vi "Configure Inputs.vi"(0 "VISA resource name":refnum<visa-resource-name>, 1 "Coupling (0: cplAC)":i32(ring) items=["cplAC", "cplDC"], 2 "Auto Range Input (T: Enable)":bool=TRUE, 3 "Enable Termination (T: Enable)":bool=TRUE, 5 "Domain (0: idAnalog)":i32(ring) items=["idAnalog", "idDigital", "idGenMon"], 7 "Channels (1)":i32=1, 9 "Connector Type (0: cXLR)":i32(ring) items=["cXLR", "cBNC", "cOptical"], 11 "error in (no error)":errorcluster, 12 "Analog Bandwidth (0: bw200kHz)":i32(ring) items=["bw200kHz", "bw50kHz", "bw25kHz"], 13 "Enable Digital Dual Connector (T: Enable)":bool=TRUE) -> (4 "VISA resource name out":refnum<visa-resource-name>, 15 "error out":errorcluster)   [LabVIEW 2014, in "Stanford Research SR1.lvlib"]
doc: "Configures the attributes for the Quick Measurement Inputs."
uses:
  Stanford Research SR1.lvlib
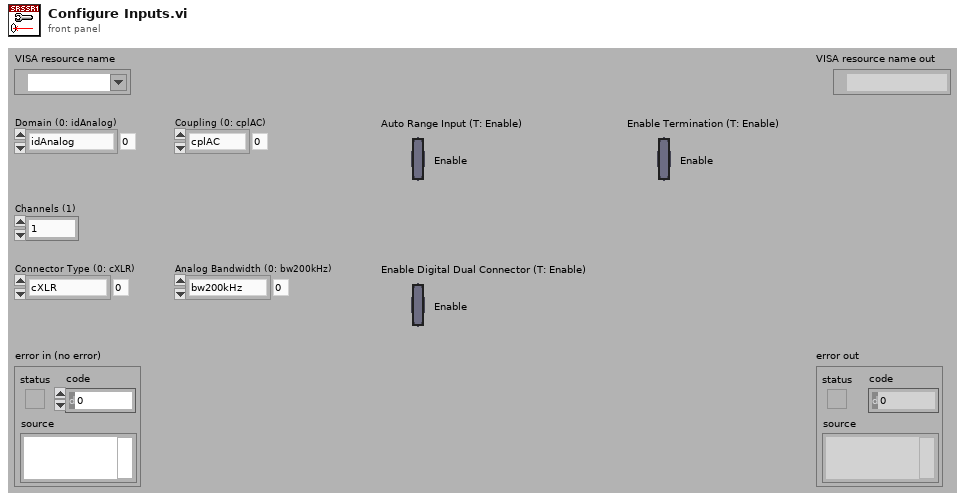
[diagram p1: front panel]
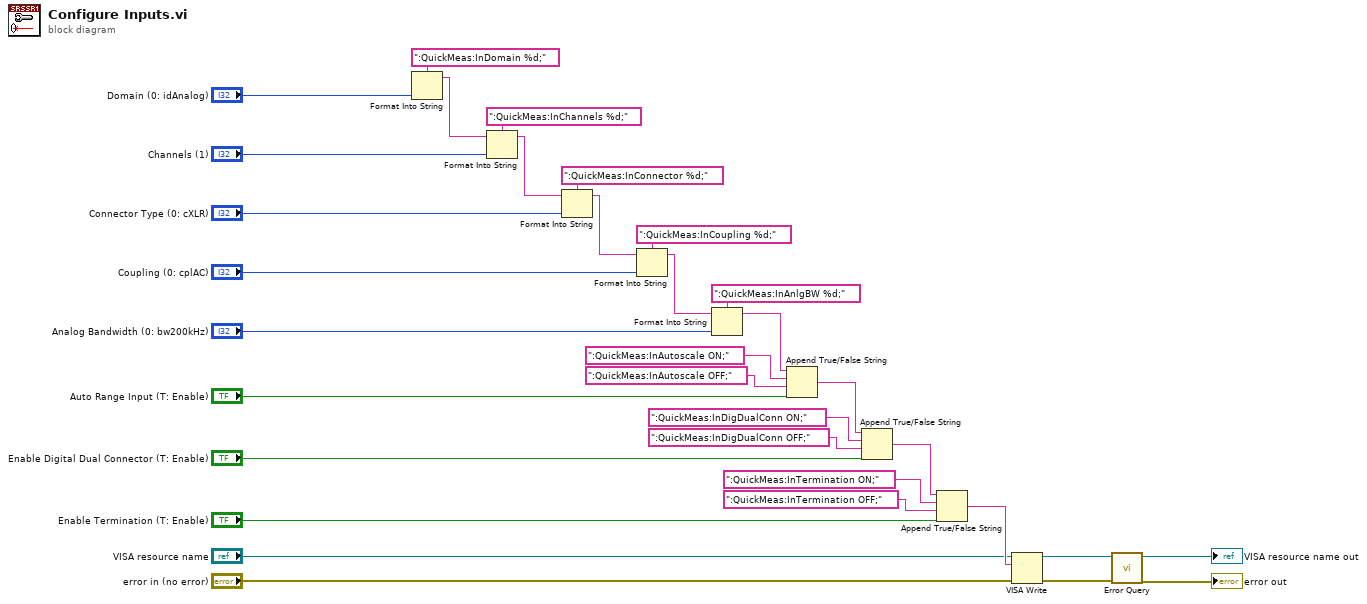
[diagram p0: block diagram]
diagram:
  n1 = Format Into String(format string=":QuickMeas:InDomain %d;", "Domain (0: idAnalog)") -> (resulting string=w31:string)  [unwired: 2 in, 1 out]
  n2 = Format Into String(format string=":QuickMeas:InChannels %d;", initial string=w31, "Channels (1)") -> (resulting string=w28:string)  [unwired: 1 in, 1 out]
  n3 = Format Into String(format string=":QuickMeas:InConnector %d;", initial string=w28, "Connector Type (0: cXLR)") -> (resulting string=w25:string)  [unwired: 1 in, 1 out]
  n4 = Format Into String(format string=":QuickMeas:InCoupling %d;", initial string=w25, "Coupling (0: cplAC)") -> (resulting string=w22:string)  [unwired: 1 in, 1 out]
  n5 = Format Into String(format string=":QuickMeas:InAnlgBW %d;", initial string=w22, "Analog Bandwidth (0: bw200kHz)") -> (resulting string=w19:string)  [unwired: 1 in, 1 out]
  n6 = Append True/False String(1:"Auto Range Input (T: Enable)", 2:":QuickMeas:InAutoscale OFF;", 3:":QuickMeas:InAutoscale ON;", 4:w19) -> (0:w15:string)
  n7 = Append True/False String(1:"Enable Digital Dual Connector (T: Enable)", 2:":QuickMeas:InDigDualConn OFF;", 3:":QuickMeas:InDigDualConn ON;", 4:w15) -> (0:w11:string)
  n8 = Append True/False String(1:"Enable Termination (T: Enable)", 2:":QuickMeas:InTermination OFF;", 3:":QuickMeas:InTermination ON;", 4:w11) -> (0:w7:string)
  n9 = VISA Write(VISA resource name="VISA resource name", write buffer=w7, error in (no error)="error in (no error)") -> (VISA resource name out=w4:refnum<visa-resource-name>, error out=w3:errorcluster)  [unwired: 1 out]
  n10 = call "Error Query.vi"("error in (no error)"=w3, "VISA resource name"=w4) -> ("error out"=→"error out":errorcluster, "VISA resource name out"=→"VISA resource name out":refnum<visa-resource-name>)  [unwired: 6 in, 2 out]
